vi "Read NI 9437 - Counter Input PWM.vi"(8 "error in":errorcluster, 11 "NI 9437 in":refnum<class "NI 9437.lvclass">) -> (0 "error out":errorcluster, 2 "channel settings":T1[](array[typedef]), 3 "NI 9437 out":refnum<class "NI 9437.lvclass">)   [LabVIEW 2020, in "Scan Engine Scripting.lvlib" / "NI 9437.lvclass"]
doc: "Returns the channel settings of a NI-9437 counter input PWM module that can be edited and then used to create a new module instance to set into a slot."
uses:
  NI 9437.lvclass
  Mode Classes/Controls/counter input pwm channel settings.ctl
  Channel Classes/PWM Input Channel/Measurement Type.ctl
  Channel Classes/PWM Input Channel/PWM Input Channel.lvclass
  Scan Engine Scripting.lvlib
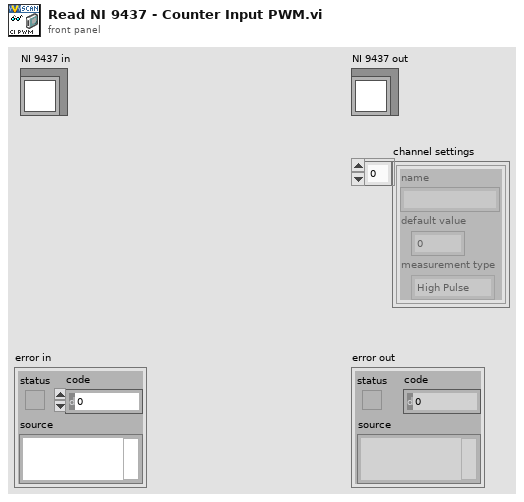
[diagram p1: front panel]
types:
  T1 = typedef "Scan Engine Scripting.lvlib/counter input pwm channel settings.ctl" = cluster{"name":string, "default value":dbl, "measurement type":T2}
  T2 = typedef "Scan Engine Scripting.lvlib/PWM Input Channel.lvclass/Measurement Type.ctl" = enum16{"High Pulse", "Low Pulse", "Most Recent"}
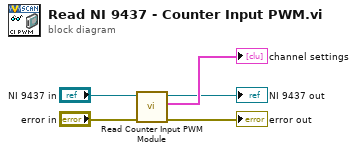
[diagram p0: block diagram]
diagram:
  n1 = call-dynamic "Read Counter Input PWM Module.vi"("error in"="error in", "module in"="NI 9437 in") -> ("error out"=→"error out":errorcluster, "channel settings"=→"channel settings":T1[], "module out"=→"NI 9437 out":refnum<class "NI 9437.lvclass">)  [unwired: 7 in]
